vi "高层函数-sequrnce.vi"() -> ()   [LabVIEW 2018]
uses:
  <vilib>/userdefined/High Color/IMAQdx.ctl
  <vilib>/vision/Image Controls.llb/IMAQ Image.ctl
  <vilib>/vision/driver/NI_Vision_Acquisition_Software.lvlib
panel:
  out "Images Out":T1[](array[typedef])
  in  "数值":i32
  out "error out":errorcluster
  in  "error in":errorcluster
  in  "Session In":T2
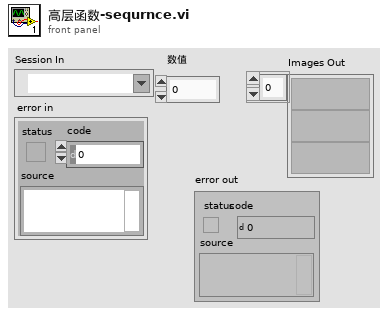
[diagram p1: front panel]
types:
  T1 = typedef "IMAQ Image.ctl" = refnum<image>
  T2 = typedef "IMAQdx.ctl" = refnum<k21>
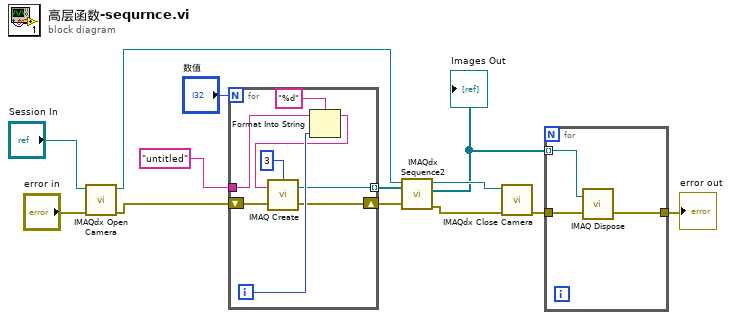
[diagram p0: block diagram]
diagram:
  n1 = call <vilib>:"IMAQdx Open Camera.vi"("error in"="error in", "Session In"="Session In") -> ("error out"=w6:errorcluster, "Session Out"=w5:T2)  [unwired: 8 in]
  n2 = for {
    N: "数值" -> [_]
    tunnel: "untitled" ("Image Name") -> [w19]
    shift-right: [w15] -> w8
    shift-left: w6 -> [w21]
    tunnel: [w14] -> w7 mode=indexing
    i -> [w18]
    n3 = Format Into String(format string="%d" ("格式字符串"), initial string=w19, w18) -> (resulting string=w16:string)  [unwired: 1 in, 1 out]
    n4 = call "IMAQ Create"("Border Size"=3, "Image Name"=w16, "error in (no error)"=w21) -> ("New Image"=w14:T1, "error out"=w15:errorcluster)  [unwired: 2 in]
  }
  n5 = call <vilib>:"IMAQdx Sequence2.vi"("error in"=w8, "Images In"=w7, "Session In"=w5) -> ("error out"=w4:errorcluster, "Images Out"=w1:T1[], "Session Out"=w3:T2)  [unwired: 6 in]
  "Images Out" <- w1
  n6 = call <vilib>:"IMAQdx Close Camera.vi"("error in"=w4, "Session In"=w3) -> ("error out"=w10:errorcluster)  [unwired: 9 in]
  n7 = for {
    tunnel: w10 -> [w24]
    tunnel: [w23] -> w2
    tunnel: w1 -> [w22] mode=indexing
    n8 = call "IMAQ Dispose"("Image"=w22, "error in (no error)"=w24) -> ("error out"=w23:errorcluster)  [unwired: 4 in]
  }
  "error out" <- w2
